vi "Min-Max Plot.vi"() -> (0 "Min Max Plot":picture)   [LabVIEW 2011]
uses:
  <vilib>/picture/cartesn2.llb/XY Plot Type.ctl
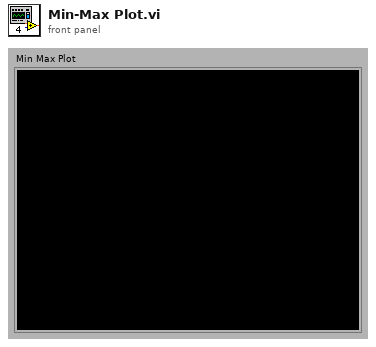
[diagram p1: front panel]
types:
  T1 = typedef "XY Plot Type.ctl" = enum16{"points", "squares", "circles", "connected points", "connected squares", "connected circles", "comb plot", "sized scatter plot", "sized-colored scatter plot", "min-max lines"}
  T2 = cluster{"plot color":u32, "xy plot type":T1, "baseline":dbl}
  T3 = typedef "LVBoundsTypeDef.ctl" = cluster{"Width":u32, "Height":u32}
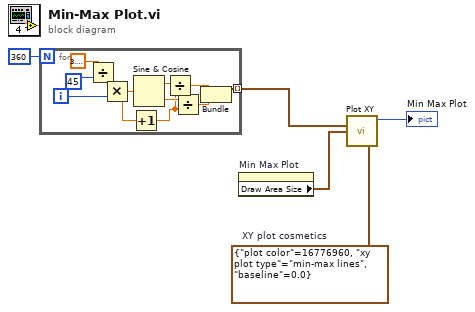
[diagram p0: block diagram]
diagram:
  w5 = T2 {"plot color"=16776960, "xy plot type"=enum."min-max lines", "baseline"=0.0}  # XY plot cosmetics
  n1 = for {
    N: 360 -> [_]
    tunnel: [w15] -> w1 mode=indexing
    i -> [w6]
    n2 = Divide(x=3.141592653589793, y=45) -> (x/y=w16:dbl)
    n3 = Multiply(x=w16, y=w6) -> (x*y=w8:dbl)
    n4 = Increment(x=w8) -> (x+1=w7:dbl)
    n5 = Sine & Cosine(0:w8) -> (1:w12:dbl, 2:w10:dbl)
    n6 = Divide(x=w12, y=w7) -> (x/y=w11:dbl)
    n7 = Divide(x=w10, y=w7) -> (x/y=w9:dbl)
    n8 = Bundle(w11, w9) -> (w15:cluster{dbl, dbl})  [unwired: 1 out]
  }
  n9 = property on="Min Max Plot" class="Pict"() -> ("Draw Area Size"=w4:T3)  [unwired: 2 in, 2 out]
  n10 = call <vilib>:"Plot XY.vi"("data"=w1, "dimensions (w,h)"=w4, "XY plot cosmetics"=w5) -> ("new picture"=→"Min Max Plot":picture)  [unwired: 3 in, 9 out]
